vi "Model Cfg Dialog.vi"(8 "error in (no error)":errorcluster, 11 "DB Ref":T2) -> (0 "error out":errorcluster)   [LabVIEW 2017]
uses:
  TagDB/Typedef/TagDB.ctl
  DEF-SineSettings.ctl
  0304f497-5d5d-4f63-a3a1-f1598543cc6a.vi
  a581869f-b58a-4321-84d3-a30686f24343.vi
  TagDB/_Support/DataAccess/_NameCacher.vi
  TagDB/_Support/DataAccess/_datatypeChecker.vi
  TagDB/_Support/DataAccess/TagDB Ref to DVR.vi
  <vilib>/Utility/error.llb/Trim Whitespace.vi
  TagDB/_Support/Error/_[error50002]Invalid DataType.vi
  TagDB/_Support/Error/_[error50000]Invalid DB REF.vi
  <vilib>/Utility/Data Type/Get Type Information.vi
  TagDB/TagDB(DEV).lvlib
panel:
  in  "CFG":T1={"frequency"=10.0, "amplitude"=1.0, "phase"=0.0, "sampling info"={"Fs"=1000.0, "#s"=1000.0}} {"frequency" format="%0.2p"; "amplitude" format="%0.2p"; "phase" format="%.2p"; "sampling info"."Fs" format="%.2p"}
  out "Cancelled?":bool
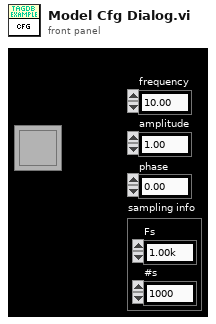
[diagram p1: front panel]
types:
  T1 = typedef "DEF-SineSettings.ctl" = cluster{"frequency":dbl, "amplitude":dbl, "phase":dbl, "sampling info":cluster{"Fs":dbl, "#s":dbl}}
  T2 = typedef "TagDB(DEV).lvlib/TagDB.ctl" = refnum<k1>
  T3 = typedef "eventvkey.ctl" = enum16{"ASCII", "Enter", "Return", "Shift", "Ctrl", "Alt", "Cmd", "Opt", "Caps", "NumLock", "Clear", "Break", "Up", "Down", "Left", "Right", "Insert", "Delete", "Home", "End", "PageUp", "PageDown", "Escape", "Help", "Pause", "ScrollLock", "F1", "F2", "F3", "F4", "F5", "F6", "F7", "F8", "F9", "F10", "F11", "F12", "F13", "F14", "F15", "F16", "F17", "F18", "F19", "F20", "F21", "F22", "F23", "F24", "Play", "VolumeUp", "VolumeDown", "Mute", "Two Byte Char"}
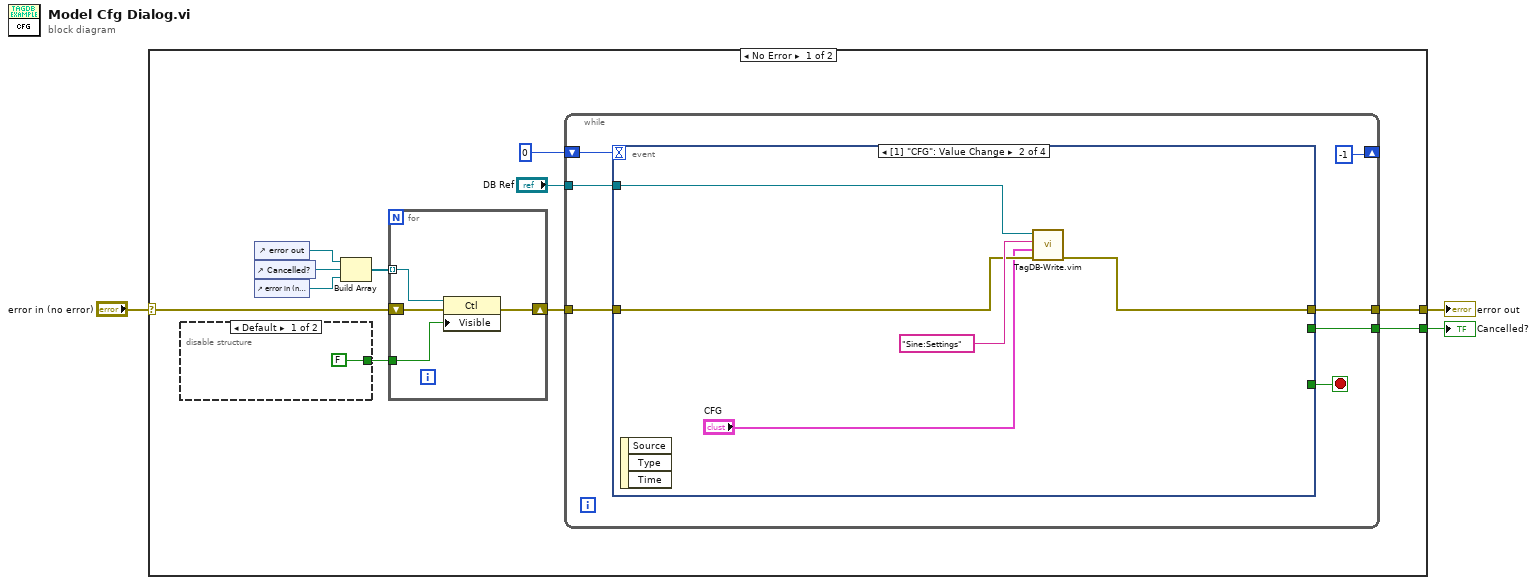
[diagram p0: block diagram]
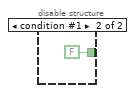
[diagram p2: hidden frame]
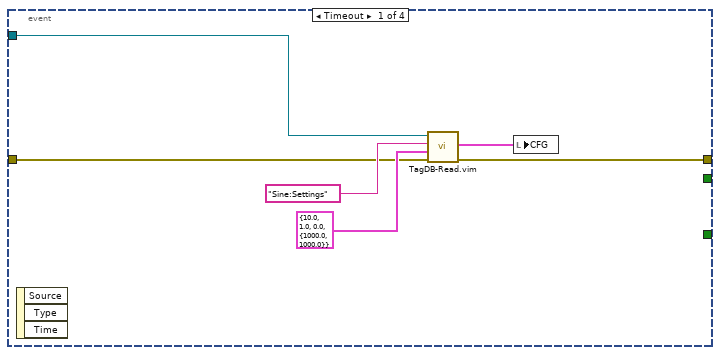
[diagram p3: hidden frame]
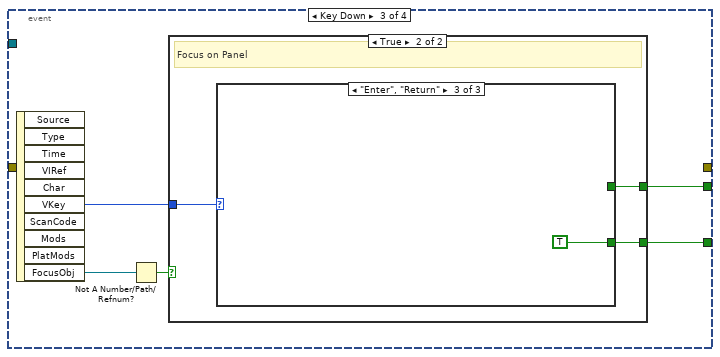
[diagram p4: hidden frame]
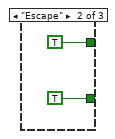
[diagram p7: hidden frame]
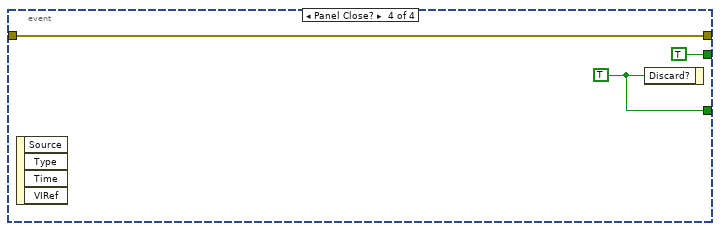
[diagram p8: hidden frame]
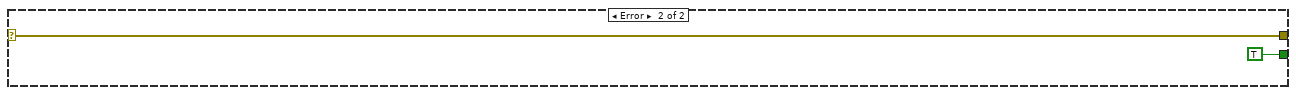
[diagram p9: hidden frame]
diagram:
  n1 = case shown="No Error" "error in (no error)" {
    selector: "error in (no error)" -> [w11 w54]
    tunnel: [w13 TRUE] -> w3
    tunnel: [w4 w54] -> w1
    frame No Error {
      n2 = disable-structure shown="Default" {
        disable-tunnel: [FALSE FALSE] -> w6
        frame condition #0 (active) {
        }
        frame condition #1 {
        }
      }
      n3 = control-ref of="error out"() -> (w8:refnum<vi>)
      n4 = control-ref of="Cancelled?"() -> (w9:refnum<vi>)
      n5 = control-ref of="error in (no error)"() -> (w10:refnum<vi>)
      n6 = Build Array(w8, w9, w10) -> (w7:refnum<vi>[])
      n7 = for {
        shift-right: [w20] -> w12
        shift-left: w11 -> [w19]
        tunnel: w7 -> [w18] mode=indexing
        tunnel: w6 -> [w17]
        n8 = property on="Property Node" class="Ctl"(reference=w18, error in=w19, "Visible"=w17) -> (error out=w20:errorcluster)  [unwired: 1 out]
      }
      n9 = while {
        shift-right: [-1] -> _
        shift-left: 0 -> [w26]
        tunnel: [w24] -> w13
        tunnel: w12 -> [w22]
        tunnel: "DB Ref" -> [w23]
        tunnel: [w21] -> w4
        stop <- w27 stop-if-true
        n10 = event shown="[1] \"CFG\": Value Change" {
          selector: _ -> [_ _ _ _]
          dyn-events: _ -> [_ _ _ _]
          timeout: w26 -> [_ _ _ _]
          tunnel: [_ _ w40 w52] -> w27
          tunnel: [_ _ w39 TRUE] -> w24
          tunnel: w23 -> [w31 w37 _ _]
          tunnel: w22 -> [w30 w36 _ w50]
          tunnel: [w29 w35 _ w50] -> w21
          event Timeout {
            n11 = event-data() -> ()  [unwired: 1 in, 3 out]
            n12 = call "TagDB-Read.vim"("error in (no error)"=w30, "Type"=T1 {"frequency"=10.0, "amplitude"=1.0, "phase"=0.0, "sampling info"={"Fs"=1000.0, "#s"=1000.0}} ("Sine Settings"), "name"="Sine:Settings", "TagDB"=w31) -> ("error out"=w29:errorcluster, "Value"=w28:T1)  [unwired: 2 in, 4 out]
            n13 = local write "CFG"(w28) -> ()
          }
          event Value Change {
            n14 = event-data() -> ()  [unwired: 1 in, 3 out]
            n15 = call "TagDB-Write.vim"("error in (no error)"=w36, "Value"="CFG", "name"="Sine:Settings", "TagDB"=w37) -> ("error out"=w35:errorcluster)  [unwired: 5 in, 2 out]
          }
          event Key Down {
            n16 = event-data() -> ("VKey"=w41:T3, "FocusObj"=w42:refnum<vi>)  [unwired: 1 in, 8 out]
            n17 = Not A Number/Path/Refnum?(number/path/refnum=w42) -> (NaN/Path/Refnum?=w43:bool)
            n18 = case shown="True" w43 {
              tunnel: w41 -> [_ w46]
              tunnel: [_ w45] -> w40
              tunnel: [_ w44] -> w39
              frame False {
                # "Focus on Obj"
              }
              frame True {
                # "Focus on Panel"
                n19 = case shown="\"Enter\", \"Return\"" w46 {
                  tunnel: [_ TRUE TRUE] -> w45
                  tunnel: [_ TRUE _] -> w44
                  frame Default {
                  }
                  frame "Escape" {
                  }
                  frame "Enter", "Return" {
                  }
                }
              }
            }
          }
          event Panel Close? {
            w52 = TRUE ("Discard?")
            n20 = event-data() -> ()  [unwired: 1 in, 4 out]
            n21 = event-data("Discard?"=w52) -> ()  [unwired: 1 in, 1 out]
          }
        }
      }
    }
    frame Error {
    }
  }
  "Cancelled?" <- w3
  "error out" <- w1
